vi "Glimpse write video header file.vi"(0 "Number of frames":u32, 1 "Sequence files handle":T2, 3 "Pixel depth\n(0=8 bit; 1= 16 bit)":u32(ring) items=["8 bits", "16 bits", "Float", "Complex", "RGB", "HSL"], 5 "error in":errorcluster, 6 "TTB Array":u32[](array[numeric]), 7 "Offsets Array":T3, 8 "Header2 file data":T1, 10 "Region width":u16, 11 "Region height":u16, 12 "Element 0 of TTB":u32, 13 "time of 1st frame, \nsec since 1/1/04":dbl format="%.2f") -> (19 "error out":errorcluster)   [LabVIEW 2016]
doc: "Closes acquisition files. Writes header file and closes it. Makes an evenly spaced time table if TTB array input is not connected; otherwise uses connected input. Set globals region width, region height, element 0 of ttb, and time of 1st frame before calling."
uses:
  Seq file v 1/Offset table.ctl
  Seq file v 1/Offset.ctl
  Seq file v 1/file number.ctl
  Sequence files handle.ctt
  Header2 file data.ctl
  Header file data.ctl
  GLIMPSE Globals.vi
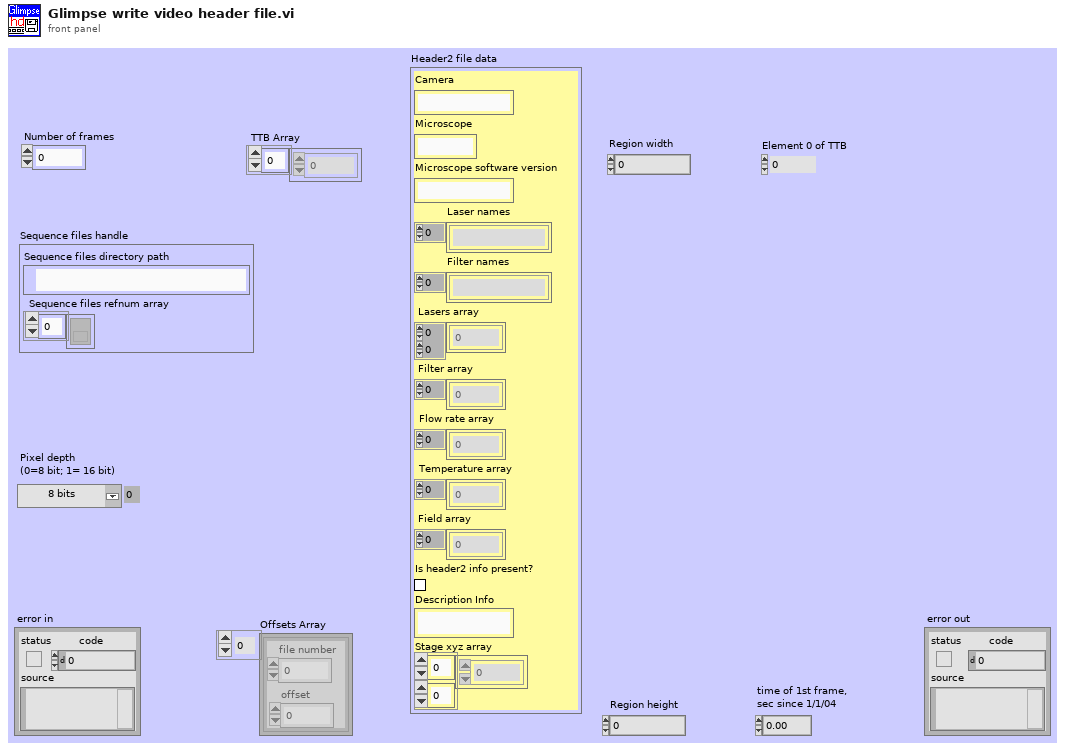
[diagram p1: front panel]
types:
  T1 = typedef "Header2 file data.ctl" = cluster{"Camera":string, "Microscope":string, "Microscope software version":string, "Laser names":string[], "Filter names":string[], "Lasers array":u16[][], "Filter array":u16[], "Flow rate array":dbl[], "Temperature array":dbl[], "Field array":u16[], "Is header2 info present?":bool, "Description Info":string, "Stage xyz array":dbl[][]}
  T2 = typedef "Sequence files handle.ctt" = cluster{"Sequence files directory path":path, "Sequence files refnum array":refnum<file>[]}
  T3 = typedef "Offset table.ctl" = cluster{"offset":T4, "file number":T5}[]
  T4 = typedef "Offset.ctl" = i32
  T5 = typedef "file number.ctl" = u8
  T6 = enum16{"open", "replace", "create", "open or create", "replace or create", "replace or create with confirmation"}
  T7 = typedef "Header file data.ctl" = cluster{"Frames Acquired":u32, "Region width":i32, "Region height":i32, "Element 0 of TTB":u32, "time of 1st frame, \nsec since 1/1/04":dbl, "TTB Array (ms)":u32[], "Offsets Array":T3, "Pixel depth":u32}
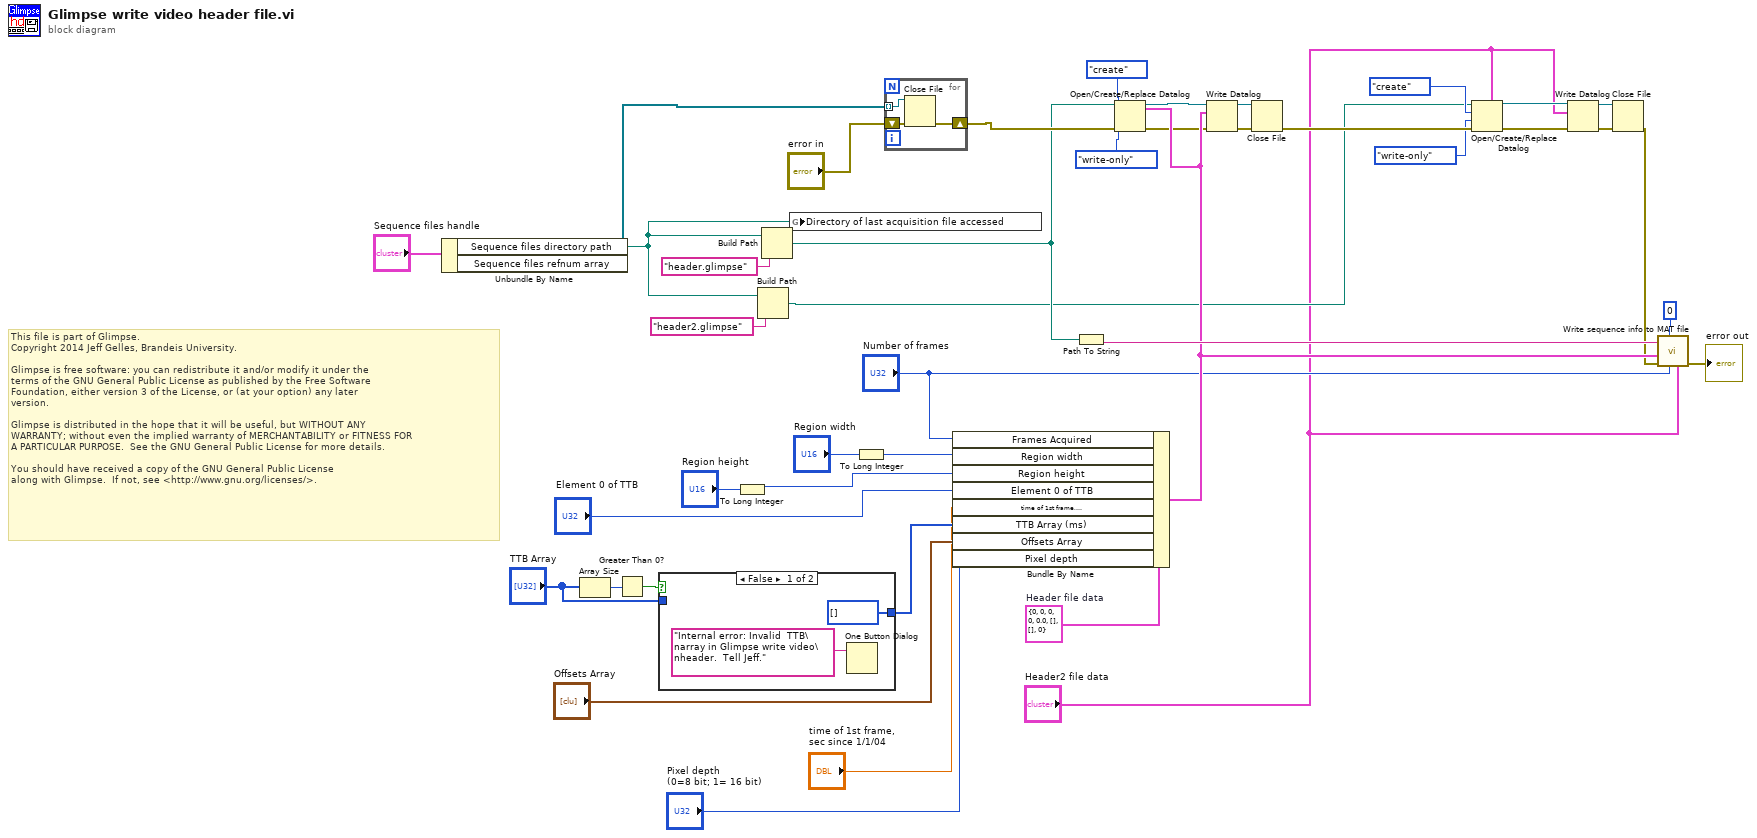
[diagram p0: block diagram]
diagram:
  w32 = T7 {"Frames Acquired"=0, "Region width"=0, "Region height"=0, "Element 0 of TTB"=0, "time of 1st frame, \nsec since 1/1/04"=0.0, "TTB Array (ms)"=[], "Offsets Array"=[], "Pixel depth"=0}  # Header file data
  # "This file is part of Glimpse. \nCopyright 2014 Jeff Gelles, Brandeis University.    \n\nGlimpse is free software: you can redistribute it and/or modify it under the \nterms of the GNU General Public License as published by the Free Software \nFoundation, either version 3 of the License, or (at your option) any later \nversion.\n\nGlimpse is distributed in the hope that it will be useful, but WITHOUT ANY \nWARRANTY; without even the implied warranty of MERCHANTABILITY or FITNESS FOR \nA PARTICULAR PURPOSE.  See the GNU General Public License for more details.\n\nYou should have received a copy of the GNU General Public License\nalong with Glimpse.  If not, see <http://www.gnu.org/licenses/>."
  n1 = Unbundle By Name("Sequence files handle") -> ("Sequence files directory path"=w12:path, "Sequence files refnum array"=w17:refnum<file>[])
  n2 = Array Size(array="TTB Array") -> (size(s)=w36:i32)
  n3 = Greater Than 0?(x=w36) -> (x > 0?=w35:bool)
  n4 = case shown="False" w35 {
    tunnel: [u32[] [] ("TTB Array") w45] -> w31
    tunnel: "TTB Array" -> [_ w45]
    frame False {
      n5 = One Button Dialog(message="Internal error: Invalid  TTB\narray in Glimpse write video\nheader.  Tell Jeff.") -> ()  [unwired: 2 out]
    }
    frame True {
    }
  }
  n6 = To Long Integer(number="Region height") -> (32bit integer=w33:i32)
  n7 = Build Path(base path=w12, name or relative path="header2.glimpse" ("search string")) -> (appended path=w3:path)
  n8 = Build Path(base path=w12, name or relative path="header.glimpse" ("search string")) -> (appended path=w24:path)
  n9 = global write "GLIMPSE Globals.vi" "Directory of last acquisition file accessed"(w12) -> ()
  n10 = To Long Integer(number="Region width") -> (32bit integer=w37:i32)
  n11 = for {
    shift-right: [w46] -> w39
    shift-left: "error in" -> [w47]
    tunnel: w17 -> [w48] mode=indexing
    n12 = Close File(refnum=w48, error in=w47) -> (error out=w46:errorcluster)  [unwired: 1 out]
  }
  n13 = Bundle By Name(cluster=w32, "Frames Acquired"="Number of frames", "Region width"=w37, "Region height"=w33, "Element 0 of TTB"="Element 0 of TTB", "time of 1st frame, \nsec since 1/1/04"="time of 1st frame, \nsec since 1/1/04", "TTB Array (ms)"=w31, "Offsets Array"="Offsets Array", "Pixel depth"="Pixel depth\n(0=8 bit; 1= 16 bit)") -> (w22:T7)
  n14 = Path To String(path=w24) -> (string=w23:string)
  n15 = Open/Create/Replace Datalog(5:w22, 8:w39, 9:enum16{"read/write", "read-only", "write-only"}."write-only" ("access (0:read/write)"), 10:T6."create" ("operation (0:open)"), 11:w24) -> (0:w10:errorcluster, 3:w9:refnum<k1>)  [unwired: 2 out]
  n16 = Write Datalog(4:w10, 6:w22, 7:w9) -> (0:w41:errorcluster, 3:w42:refnum<k1>)
  n17 = Close File(refnum=w42, error in=w41) -> (error out=w6:errorcluster)  [unwired: 1 out]
  n18 = Open/Create/Replace Datalog(5:"Header2 file data", 8:w6, 9:enum16{"read/write", "read-only", "write-only"}."write-only" ("access (0:read/write)"), 10:T6."create" ("operation (0:open)"), 11:w3) -> (0:w8:errorcluster, 3:w7:refnum<k1>)  [unwired: 2 out]
  n19 = Write Datalog(4:w8, 6:"Header2 file data", 7:w7) -> (0:w16:errorcluster, 3:w15:refnum<k1>)
  n20 = Close File(refnum=w15, error in=w16) -> (error out=w14:errorcluster)  [unwired: 1 out]
  n21 = call "Write sequence info to MAT file.vi"("Header2 file data"="Header2 file data", "Number of frames"="Number of frames", "first frame number"=u32 0, "error in"=w14, "Header file data"=w22, "Movie file name"=w23) -> ("error out"=→"error out":errorcluster)  [unwired: 1 in, 4 out]
